vi "Actor Core.vi"(8 "error in":errorcluster, 11 "Abstruct View in":refnum<class "Abstruct View.lvclass">) -> (0 "error out":errorcluster, 3 "Actor out":refnum<class "Actor.lvclass">)   [LabVIEW 2020, in "Abstruct View.lvlib" / "Abstruct View.lvclass"]
doc: "(<B>Filename</B>: Actor Framework.lvlib:Actor.lvclass:Actor Core.vi)\n\nReceives messages to the actor, reacts to them, and initiates any error handling that may shut the actor down.\n\nDescendant classes may override this VI to append parallel tasks for the actor to complete while it handles messages. Overrides use the Call Parent Class Method node."
uses:
  Abstruct View.lvclass
  <vilib>/ActorFramework/Actor/Actor.lvclass
  Abstruct View.lvclass/Abstruct View.ctl
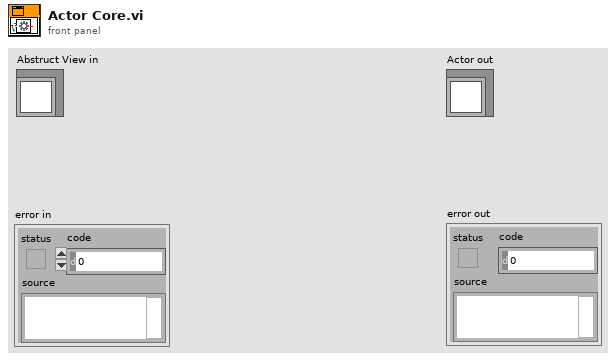
[diagram p1: front panel]
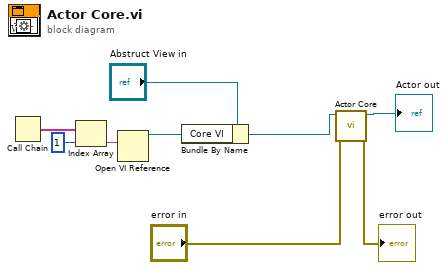
[diagram p0: block diagram]
diagram:
  n1 = Call Chain() -> (call chain=w4:string[])
  n2 = Index Array(array=w4, index=1) -> (element=w2:string)
  n3 = Open VI Reference(vi path=w2) -> (vi reference=w1:refnum<vi>)  [unwired: 5 in, 1 out]
  n4 = Bundle By Name(cluster="Abstruct View in", "Core VI"=w1) -> (w5:refnum<class "Abstruct View.lvclass">)
  n5 = call-parent "Actor Core.vi"("error in"="error in", "Actor in"=w5) -> ("error out"=→"error out":errorcluster, "Actor out"=→"Actor out":refnum<class "Actor.lvclass">)  [unwired: 8 in]
